vi "PPMS temp status.vi"(0 "GPIB address":string="15", 1 "Transmit Mode (0)":T1(ring), 2 "error in (no error)":errorcluster) -> (5 "Status bits 0-3":i32)   [LabVIEW 2017]
doc: "This VI returns the temperature status of the chamber. Temperature Stable? will be true only if the PPMS unit reports stable for the temperature and the temperature is within .5% of the set temperature. The Temperature Status string mimics the display as it is seen on the PPMS LCD readout. Status bits 0-3 returns the decimal representation of the four bits containing the status, which can be used for low level or numerical checks. It is a number 0-15 ."
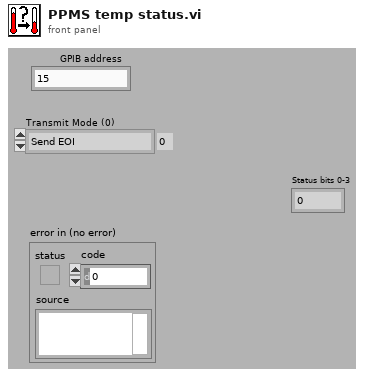
[diagram p1: front panel]
types:
  T1 = enum16{"Send EOI", "append CR w/ EOI", "append LF w/ EOI", "append CR LF w/ EOI", "append CR w/o EOI", "append LF w/o EOI", "append CR LF w/o EOI", "do not send EOI"}
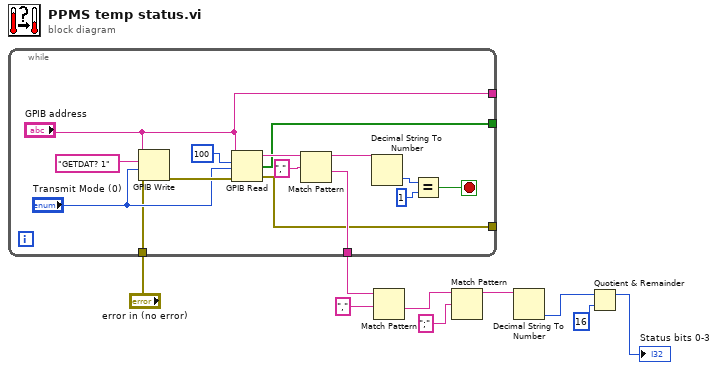
[diagram p0: block diagram]
diagram:
  n1 = while {
    tunnel: [w15] -> w9
    tunnel: ["GPIB address"] -> _
    tunnel: [w14] -> _
    tunnel: "error in (no error)" -> [w11]
    tunnel: [w10] -> _
    stop <- w16 stop-if-true
    n2 = GPIB Write(0:"GPIB address", 1:"GETDAT? 1", 2:"Transmit Mode (0)", 3:w11) -> (6:w23:errorcluster)  [unwired: 1 in, 1 out]
    n3 = GPIB Read(0:"GPIB address", 1:100, 2:"Transmit Mode (0)", 3:w23) -> (5:w21:string, 6:w14:bool[], 7:w10:errorcluster)  [unwired: 1 in]
    n4 = Match Pattern(string=w21, regular expression=",") -> (before substring=w19:string, after substring=w15:string)  [unwired: 1 in, 2 out]
    n5 = Decimal String To Number(string=w19) -> (number=w18:i32)  [unwired: 2 in, 1 out]
    n6 = Equal?(x=w18, y=1) -> (x = y?=w16:bool)
  }
  n7 = Match Pattern(string=w9, regular expression=",") -> (after substring=w7:string)  [unwired: 1 in, 3 out]
  n8 = Match Pattern(string=w7, regular expression=";") -> (before substring=w5:string)  [unwired: 1 in, 3 out]
  n9 = Decimal String To Number(string=w5) -> (number=w4:i32)  [unwired: 2 in, 1 out]
  n10 = Quotient & Remainder(x=w4, y=16) -> (x-y*floor(x/y)=→"Status bits 0-3":i32)  [unwired: 1 out]
